vi "Set Windows Shortcut Properties.vi"(4 "error in":errorcluster, 6 "Shortcut Options":T1, 7 "IWshRuntimeLibrary.IWshShortcut":refnum<k7>) -> (0 "error out":errorcluster, 3 "dup IWshRuntimeLibrary.IWshShortcut":refnum<k7>)   [LabVIEW 2011]
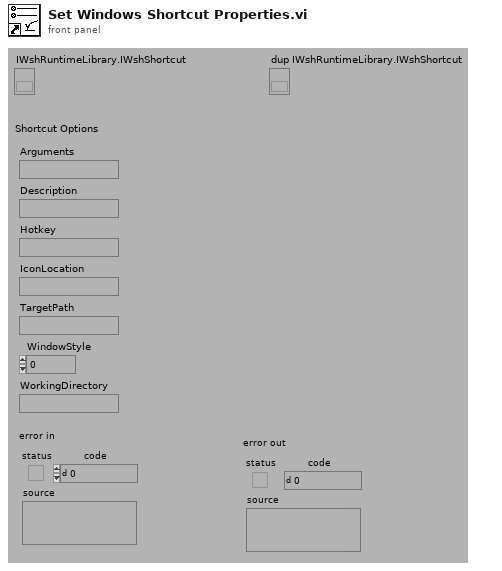
[diagram p1: front panel]
types:
  T1 = cluster{"Arguments":string, "Description":string, "Hotkey":string, "IconLocation":string, "TargetPath":string, "WindowStyle":i32, "WorkingDirectory":string}
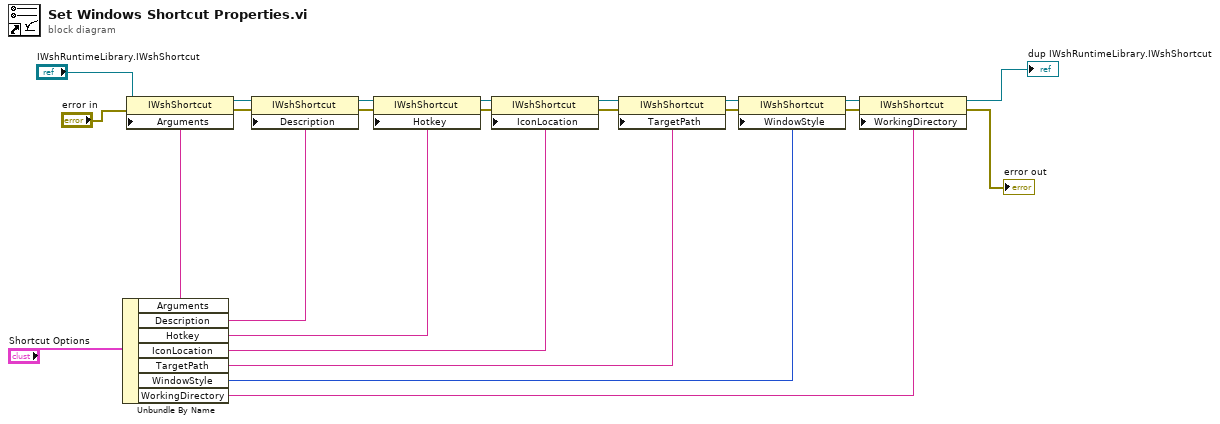
[diagram p0: block diagram]
diagram:
  n1 = Unbundle By Name("Shortcut Options") -> ("Arguments"=w16:string, "Description"=w17:string, "Hotkey"=w18:string, "IconLocation"=w19:string, "TargetPath"=w20:string, "WindowStyle"=w21:i32, "WorkingDirectory"=w22:string)
  n2 = property class="IWshShortcut"(reference="IWshRuntimeLibrary.IWshShortcut", error in="error in", "Arguments"=w16) -> (reference out=w3:refnum<k7>, error out=w4:errorcluster)
  n3 = property class="IWshShortcut"(reference=w3, error in=w4, "Description"=w17) -> (reference out=w5:refnum<k7>, error out=w6:errorcluster)
  n4 = property class="IWshShortcut"(reference=w5, error in=w6, "Hotkey"=w18) -> (reference out=w7:refnum<k7>, error out=w8:errorcluster)
  n5 = property class="IWshShortcut"(reference=w7, error in=w8, "IconLocation"=w19) -> (reference out=w13:refnum<k7>, error out=w14:errorcluster)
  n6 = property class="IWshShortcut"(reference=w13, error in=w14, "TargetPath"=w20) -> (reference out=w9:refnum<k7>, error out=w10:errorcluster)
  n7 = property class="IWshShortcut"(reference=w9, error in=w10, "WindowStyle"=w21) -> (reference out=w11:refnum<k7>, error out=w12:errorcluster)
  n8 = property class="IWshShortcut"(reference=w11, error in=w12, "WorkingDirectory"=w22) -> (reference out=→"dup IWshRuntimeLibrary.IWshShortcut":refnum<k7>, error out=→"error out":errorcluster)
